vi "control_lasers_ETL3_mirror.vi"() -> ()   [LabVIEW 2017]
uses:
  <vilib>/DAQmx/write.llb/DAQmx Write (Analog 1D DBL NChan 1Samp).vi
  <vilib>/DAQmx/create/channels.llb/DAQmx Create Channel (AO-Voltage-Basic).vi
  <vilib>/DAQmx/miscellaneous.llb/DAQmx Fill In Error Info.vi
panel:
  in  "Y multiplier":dbl=1.0
  in  "X multiplier":dbl=-1.0
  in  "Y (v)":dbl(slide) min=-10.0 max=10.0 step=0.01 scale=-10.0..10.0
  in  "X (v)":dbl(slide) min=-10.0 max=10.0 step=0.01 scale=-10.0..10.0
  in  "Combined Movement (v)\nEquation: X * X Multiplier + Y * Y Multiplier":dbl(slide) min=-10.0 max=10.0 step=0.01 scale=-10.0..10.0
  out "Focal Distance (um) 2":dbl
  out "Diopter 2":dbl
  in  "ETL3 (v) [4.76V allows light passing through unaltered]":dbl(slide)=4.76 min=-10.0 max=10.0 step=0.01 scale=-10.0..10.0
  in  "Blanking (0-10v)":dbl=10.0
  in  "561 (0-10v)":dbl
  in  "514 (0-10v)":dbl
  in  "488 (0-10v)":dbl
  in  "445 (0-10v)":dbl
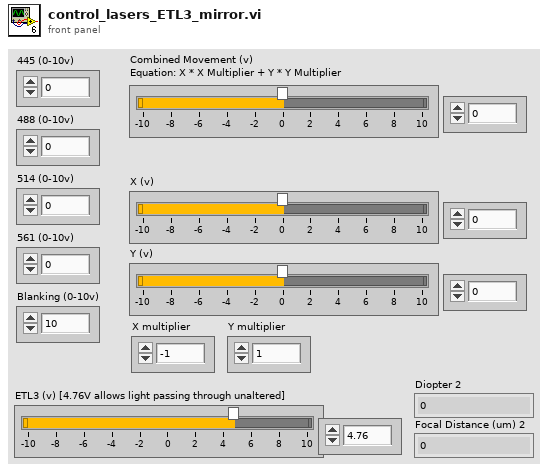
[diagram p1: front panel]
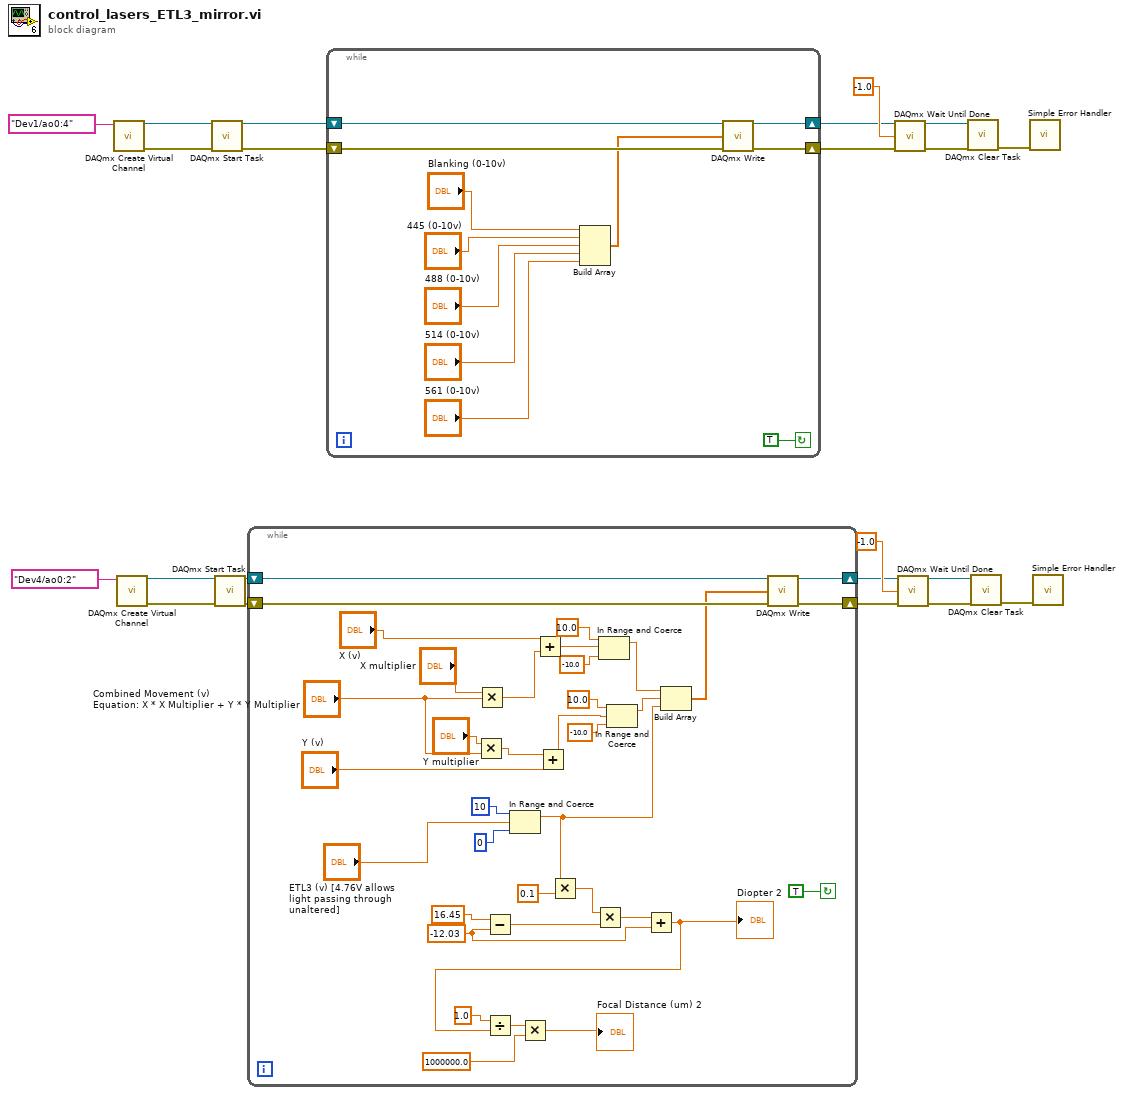
[diagram p0: block diagram]
diagram:
  n1 = call-poly <vilib>:"DAQmx Create Virtual Channel.vi"("physical channels"=tag "Dev1/ao0:4") -> ("task out"=w15:refnum<k21>, "error out"=w14:errorcluster)  [unwired: 13 in]
  n2 = call-poly <vilib>:"DAQmx Create Virtual Channel.vi"("physical channels"=tag "Dev4/ao0:2") -> ("task out"=w4:refnum<k21>, "error out"=w3:errorcluster)  [unwired: 13 in]
  n3 = call <vilib>:"DAQmx Start Task.vi"("task/channels in"=w15, "error in"=w14) -> ("task out"=w17:refnum<k21>, "error out"=w16:errorcluster)  [unwired: 12 in]
  n4 = call <vilib>:"DAQmx Start Task.vi"("task/channels in"=w4, "error in"=w3) -> ("task out"=w6:refnum<k21>, "error out"=w5:errorcluster)  [unwired: 12 in]
  n5 = while {
    shift-right: [w56] -> w1
    shift-left: w6 -> [w58]
    shift-right: [w55] -> w2
    shift-left: w5 -> [w57]
    stop <- TRUE continue-if-true
    w32 = -12.03 ("x")
    n6 = Multiply(x="Y multiplier", y="Combined Movement (v)\nEquation: X * X Multiplier + Y * Y Multiplier") -> (x*y=w43:dbl)
    n7 = Multiply(x="X multiplier", y="Combined Movement (v)\nEquation: X * X Multiplier + Y * Y Multiplier") -> (x*y=w52:dbl)
    n8 = Subtract(x=16.45 ("y"), y=w32) -> (x-y=w34:dbl)
    n9 = In Range and Coerce(upper limit=10, x="ETL3 (v) [4.76V allows light passing through unaltered]", lower limit=0) -> (coerced(x)=w31:dbl)  [unwired: 1 out]
    n10 = Add(x="X (v)", y=w52) -> (x+y=w51:dbl)
    n11 = Add(x=w43, y="Y (v)") -> (x+y=w45:dbl)
    n12 = Multiply(x=w31, y=0.1) -> (x*y=w35:dbl)
    n13 = Multiply(x=w35, y=w34) -> (x*y=w33:dbl)
    n14 = In Range and Coerce(upper limit=10.0, x=w51, lower limit=-10.0) -> (coerced(x)=w48:dbl)  [unwired: 1 out]
    n15 = In Range and Coerce(upper limit=10.0, x=w45, lower limit=-10.0) -> (coerced(x)=w44:dbl)  [unwired: 1 out]
    n16 = Add(x=w33, y=w32) -> (x+y=w23:dbl)
    "Diopter 2" <- w23
    n17 = Divide(x=1.0, y=w23) -> (x/y=w41:dbl)
    n18 = Multiply(x=w41, y=1000000.0) -> (x*y=→"Focal Distance (um) 2":dbl)
    n19 = Build Array(w48, w44, w31) -> (w54:dbl[])
    n20 = call-poly <vilib>:"DAQmx Write.vi"("task/channels in"=w58, "data"=w54, "error in"=w57) -> ("task out"=w56:refnum<k21>, "error out"=w55:errorcluster)  [unwired: 10 in, 1 out]
  }
  n21 = while {
    shift-right: [w67] -> w12
    shift-left: w17 -> [w69]
    shift-right: [w66] -> w13
    shift-left: w16 -> [w68]
    stop <- TRUE continue-if-true
    n22 = Build Array("Blanking (0-10v)", "445 (0-10v)", "488 (0-10v)", "514 (0-10v)", "561 (0-10v)") -> (w59:dbl[])
    n23 = call-poly <vilib>:"DAQmx Write.vi"("task/channels in"=w69, "data"=w59, "error in"=w68) -> ("task out"=w67:refnum<k21>, "error out"=w66:errorcluster)  [unwired: 10 in, 1 out]
  }
  n24 = call <vilib>:"DAQmx Wait Until Done.vi"("task/channels in"=w12, "timeout (sec)"=-1.0, "error in"=w13) -> ("task out"=w21:refnum<k21>, "error out"=w20:errorcluster)  [unwired: 11 in]
  n25 = call <vilib>:"DAQmx Wait Until Done.vi"("task/channels in"=w1, "timeout (sec)"=-1.0, "error in"=w2) -> ("task out"=w10:refnum<k21>, "error out"=w9:errorcluster)  [unwired: 11 in]
  n26 = call <vilib>:"DAQmx Clear Task.vi"("task in"=w21, "error in"=w20) -> ("error out"=w22:errorcluster)  [unwired: 13 in]
  n27 = call <vilib>:"DAQmx Clear Task.vi"("task in"=w10, "error in"=w9) -> ("error out"=w11:errorcluster)  [unwired: 13 in]
  n28 = call <vilib>:"Simple Error Handler.vi"("error in (no error)"=w22) -> ()  [unwired: 4 in, 5 out]
  n29 = call <vilib>:"Simple Error Handler.vi"("error in (no error)"=w11) -> ()  [unwired: 4 in, 5 out]
